vi "Main.vi"() -> ()   [LabVIEW 2019]
doc: "The myRIO Project template acquires acceleration data from the onboard accelerometer and displays the changes of acceleration values in a waveform chart."
uses:
  <vilib>/myRIO/Instrument Drivers/Onboard IO/DIO/typedefs/DIO Reference.ctl
  <vilib>/myRIO/Common/Instrument Driver Framework/Utilities/typedefs/myRIO Generic Hardware Reference.ctl
  <vilib>/myRIO/Common/Instrument Driver Framework/Utilities/typedefs/Hardware Version Enum.ctl
  <vilib>/myRIO/Common/Instrument Driver Framework/Utilities/typedefs/myRIO v1.0 Reference.ctl
  <vilib>/myRIO/Common/Instrument Driver Framework/Utilities/typedefs/Generic FPGA Reference.ctl
  <vilib>/myRIO/Common/Instrument Driver Framework/myRIO v1.0/DIO/typedefs/DIO Channels List.ctl
  <vilib>/myRIO/Common/Instrument Driver Framework/myRIO v1.0/DIO/typedefs/DIO Channels Enum.ctl
  <vilib>/userDefined/High Color/nirio_resource_hc.ctl
  <vilib>/myRIO/Common/Instrument Driver Framework/Utilities/vis/Is FPGA Ref Available.vi
  <vilib>/myRIO/Common/Instrument Driver Framework/myRIO v1.0/DIO/vis/myRIO v1.1 Open DIO.vi
  <vilib>/myRIO/Instrument Drivers/Onboard IO/DIO/vis/Write.vi
  <vilib>/myRIO/Common/Instrument Driver Framework/Utilities/vis/Validate Channels.vi
  <vilib>/myRIO/Common/Instrument Driver Framework/myRIO v1.0/DIO/vis/myRIO v1.0 Reserve DIO.vi
  <vilib>/myRIO/Common/Instrument Driver Framework/myRIO v1.0/UART/vis/myRIO v1.0 Close UART.vi
  <vilib>/myRIO/Common/Instrument Driver Framework/myRIO v1.0/Resource Manager/vis/myRIO v1.0 Reserve Channel List.vi
  <vilib>/myRIO/Common/Instrument Driver Framework/myRIO v1.0/DIO/vis/myRIO v1.0 Build MUX Configuration DIO.vi
  <vilib>/myRIO/Common/Instrument Driver Framework/myRIO v1.0/Resource Manager/vis/myRIO v1.0 Reserve Channel.vi
  <vilib>/myRIO/Common/Instrument Driver Framework/myRIO v1.0/Resource Manager/vis/myRIO v1.0 Unreserve Channel.vi
  <vilib>/myRIO/Common/Instrument Driver Framework/myRIO v1.0/Resource Manager/vis/myRIO v1.0 Create Configuration List.vi
  <vilib>/myRIO/Common/Instrument Driver Framework/myRIO v1.0/Resource Manager/vis/myRIO v1.0 Build Mutex Name.vi
  <vilib>/Utility/VariantDataType/GetNumericInfo.vi
  <vilib>/Utility/error.llb/Error Cluster From Error Code.vi
  <vilib>/myRIO/Common/Instrument Driver Framework/myRIO v1.0/myRIO v1.1 Open.vi
  <vilib>/myRIO/Common/Instrument Driver Framework/Utilities/vis/IO Manager.vi
  <vilib>/myRIO/Common/Instrument Driver Framework/Utilities/vis/Configuration Manager.vi
  <vilib>/myRIO/Common/Instrument Driver Framework/myRIO v1.0/Resource Manager/vis/myRIO v1.0 Configure IO.vi
  <vilib>/myRIO/Common/Instrument Driver Framework/myRIO v1.0/myRIO v1.0 Close.vi
  <vilib>/myRIO/Common/Instrument Driver Framework/myRIO v1.0/DIO/vis/myRIO v1.0 Write DIO.vi
  <vilib>/myRIO/Common/Instrument Driver Framework/Utilities/vis/FPGA Ref Manager.vi
  <vilib>/myRIO/Common/Instrument Driver Framework/myRIO v1.0/myRIO v1.0 Reset FPGA.vi
  <vilib>/myRIO/Common/Instrument Driver Framework/myRIO v1.0/IRQ/vis/myRIO v1.0 IRQ Info FGV.vi
  <vilib>/myRIO/Common/Instrument Driver Framework/myRIO v1.0/IRQ/vis/myRIO v1.0 Timer IRQ Info FGV.vi
  <vilib>/myRIO/Common/Instrument Driver Framework/myRIO v1.0/IRQ/vis/myRIO v1.0 ISR Agent.vi
  <vilib>/myRIO/Instrument Drivers/Utilities/vis/Reset Index.vi
  <vilib>/myRIO/Common/Instrument Driver Framework/myRIO v1.0/Resource Manager/vis/myRIO v1.0 Block Write Resource Manager.vi
  <vilib>/myRIO/Express VI/Onboard IO/DO/DO Express VI.xnode
  <vilib>/myRIO/Instrument Drivers/Onboard IO/DIO/vis/myRIO DIO Open.xnode
  <vilib>/myRIO/Instrument Drivers/Utilities/Utilities.lvlib
  <vilib>/myRIO/Instrument Drivers/Onboard IO/DIO/DIO.lvlib
panel:
  out "Polar Plot":picture
  in  "stop":bool
  in  "seperation factor":i32(slide) scale=1.0..12.0
  in  "Phase Const":i64(slide) scale=0.0..360.0
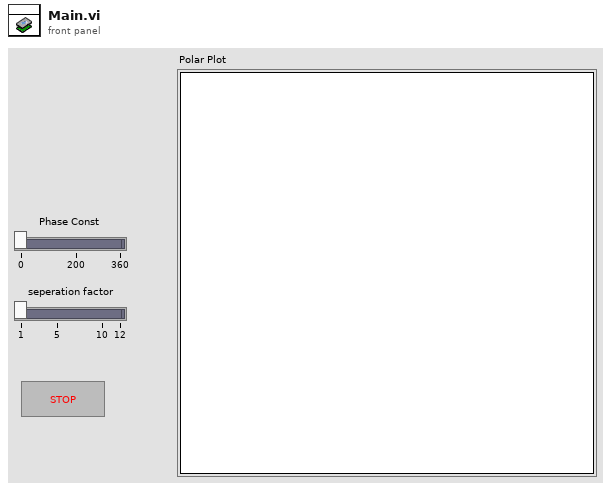
[diagram p1: front panel]
types:
  T1 = typedef "DIO.lvlib/DIO Reference.ctl" = cluster{"myRIO Reference":T2, "DIO Channels List":T6}
  T2 = typedef "myRIO Generic Hardware Reference.ctl" = cluster{"myRIO Model":T3, "myRIO Hardware Reference":T4}
  T3 = typedef "Hardware Version Enum.ctl" = enum16{"Unknown", "myRIO-1900", "myRIO-1950", "roboRIO", "NI ELVIS RIO CM", "ELVIS III"}
  T4 = typedef "myRIO v1.0 Reference.ctl" = cluster{"Generic FPGA Reference":T5, "Allow multiple opens":bool}
  T5 = typedef "Generic FPGA Reference.ctl" = refnum<k20>
  T6 = typedef "DIO Channels List.ctl" = T7[]
  T7 = typedef "DIO Channels Enum.ctl" = enum16{"Not Connected", "C/DIO0", "C/DIO1", "C/DIO2", "C/DIO3", "C/DIO4", "C/DIO5", "C/DIO6", "C/DIO7", "A/DIO0", "A/DIO1", "A/DIO2", "A/DIO3", "A/DIO4", "A/DIO5", "A/DIO6", "A/DIO7", "A/DIO8", "A/DIO9", "A/DIO10", "A/DIO11", "A/DIO12", "A/DIO13", "A/DIO14", "A/DIO15", "A/DIO16", "A/DIO17", "A/DIO18", "A/DIO19", "B/DIO0", "B/DIO1", "B/DIO2", "B/DIO3", "B/DIO4", "B/DIO5", "B/DIO6", "B/DIO7", "B/DIO8", "B/DIO9", "B/DIO10", "B/DIO11", "B/DIO12", "B/DIO13", "B/DIO14", "B/DIO15", "B/DIO16", "B/DIO17", "B/DIO18", "B/DIO19", "LED0", "LED1", "LED2", "LED3", "Button0", "DIO/DIO0", "DIO/DIO1", "DIO/DIO2", "DIO/DIO3", "DIO/DIO4", "DIO/DIO5", "DIO/DIO6", "DIO/DIO7", "DIO/DIO8", "DIO/DIO9", "SPI/CS0", "SPI/CS1", "SPI/CS2", "SPI/CS3", "LED RADIO (Green)", "LED RADIO (Red)", "LED COMM (Green)", "LED COMM (Red)", "LED MODE (Green)", "LED MODE (Red)"}
  T8 = typedef "nirio_resource_hc.ctl" = tag
  T9 = typedef "LVBoundsTypeDef.ctl" = cluster{"Width":u32, "Height":u32}
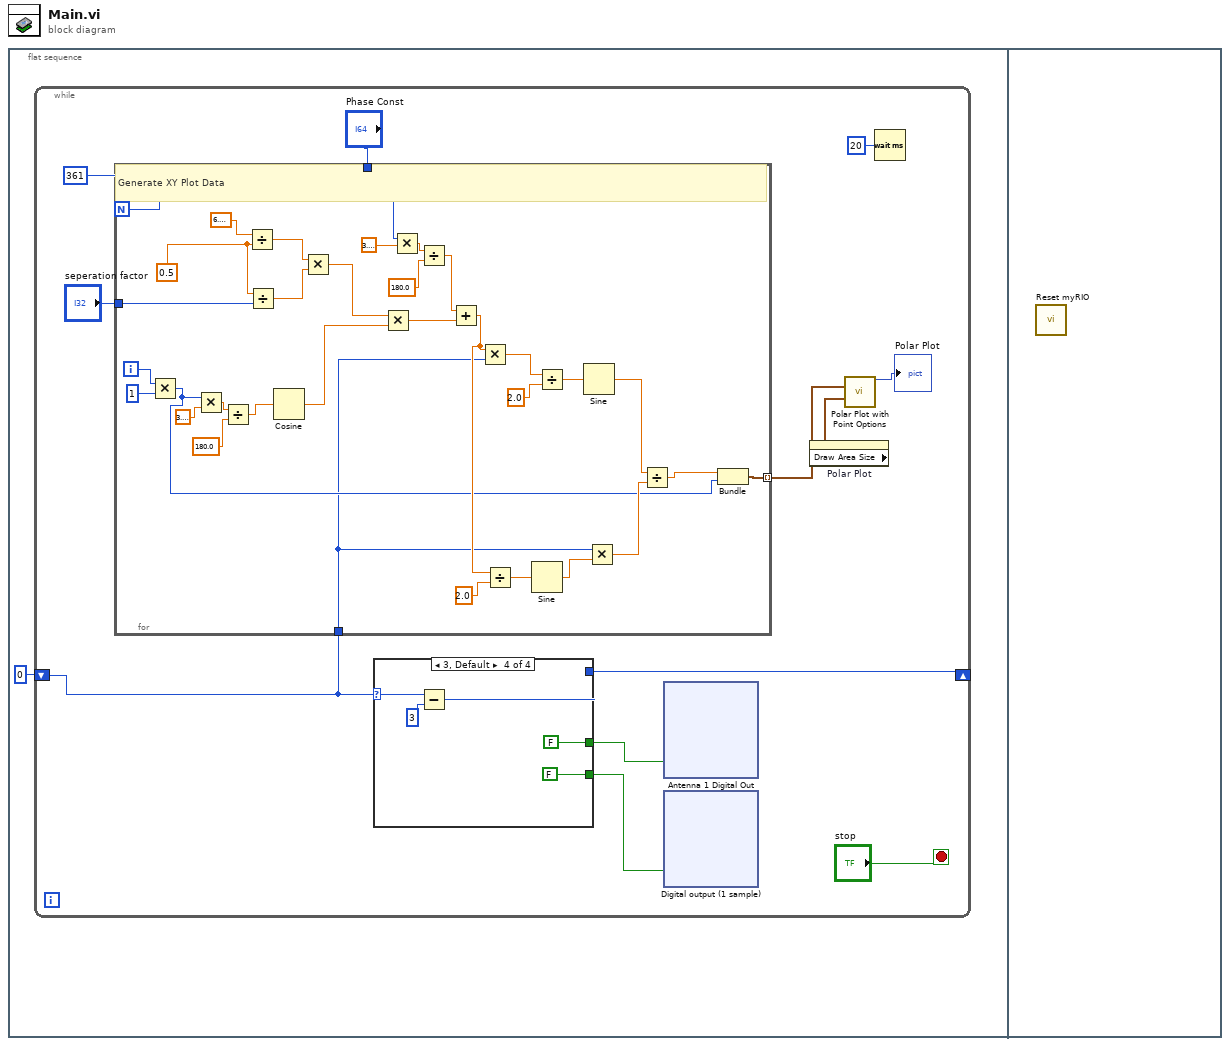
[diagram p0: block diagram]
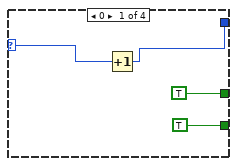
[diagram p2: hidden frame]
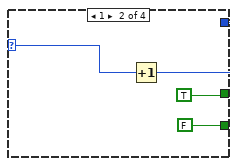
[diagram p3: hidden frame]
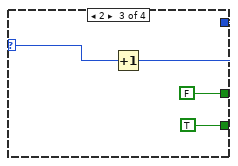
[diagram p4: hidden frame]
diagram:
  n1 = flat-sequence {
    frame #0 {
      n2 = while {
        shift-right: [w7] -> _
        shift-left: 0 -> [w4]
        stop <- "stop" stop-if-true
        n3 = for {
          N: 361 -> [_]
          tunnel: [w113] -> w10 mode=indexing
          tunnel: "seperation factor" -> [w103]
          tunnel: "Phase Const" -> [w102]
          tunnel: w4 -> [w101]
          i -> [w114]
          w122 = 0.5 ("Labda")
          # "Generate XY Plot Data"
          n4 = Multiply(x=w114, y=1) -> (x*y=w104:i32)
          n5 = Multiply(x=w104, y=3.141592653589793) -> (x*y=w126:dbl)
          n6 = Divide(x=w126, y=180.0) -> (x/y=w127:dbl)
          n7 = Divide(x=6.283185307179586, y=w122) -> (x/y=w123:dbl)
          n8 = Divide(x=w122, y=w103) -> (x/y=w124:dbl)
          n9 = Cosine(x=w127) -> (cos(x)=w125:dbl)
          n10 = Multiply(x=w123, y=w124) -> (x*y=w128:dbl)
          n11 = Multiply(x=w128, y=w125) -> (x*y=w131:dbl)
          n12 = Multiply(x=w102, y=3.141592653589793) -> (x*y=w129:dbl)
          n13 = Divide(x=w129, y=180.0) -> (x/y=w130:dbl)
          n14 = Add(x=w130, y=w131) -> (x+y=w105:dbl)
          n15 = Multiply(x=w105, y=w101) -> (x*y=w112:dbl)
          n16 = Divide(x=w105, y=2.0) -> (x/y=w111:dbl)
          n17 = Sine(x=w111) -> (sin(x)=w109:dbl)
          n18 = Divide(x=w112, y=2.0) -> (x/y=w132:dbl)
          n19 = Sine(x=w132) -> (sin(x)=w108:dbl)
          n20 = Multiply(x=w101, y=w109) -> (x*y=w107:dbl)
          n21 = Divide(x=w108, y=w107) -> (x/y=w106:dbl)
          n22 = Bundle(w106, w104) -> (w113:cluster{dbl, i32})  [unwired: 1 in]
        }
        n23 = case shown="3, Default" w4 {
          selector: w4 -> [w87 w91 w95 w100]
          tunnel: [w86 w90 w94 w98] -> w7
          tunnel: [TRUE TRUE FALSE FALSE] -> w3
          tunnel: [TRUE FALSE TRUE FALSE] -> w2
          frame 0 {
            n24 = Increment(x=w87) -> (x+1=w86:i32)
          }
          frame 1 {
            n25 = Increment(x=w91) -> (x+1=w90:i32)
          }
          frame 2 {
            n26 = Increment(x=w95) -> (x+1=w94:i32)
          }
          frame 3, Default {
            n27 = Subtract(x=w100, y=3) -> (x-y=w98:i32)
          }
        }
        n28 = xnode "Antenna 1 Digital Out"("A/DIO0 (Pin 11)"=w3) -> ()  [unwired: 1 in, 1 out]
        n29 = xnode "Digital output (1 sample)"("A/DIO1 (Pin 13)"=w2) -> ()  [unwired: 1 in, 1 out]
        n30 = property on="Polar Plot" class="Pict"() -> ("Draw Area Size"=w11:T9)  [unwired: 2 in, 2 out]
        n31 = call <vilib>:"Polar Plot with Point Options.vi"("data array [mag, phase (deg)]"=w10, "dimensions (w,h)"=w11) -> ("new picture"=→"Polar Plot":picture)  [unwired: 13 in]
        n32 = Wait (ms)(milliseconds to wait=u32 20) -> ()  [unwired: 1 out]
      }
    }
    frame #1 {
      n33 = call <vilib>:"Reset myRIO.vi"() -> ()  [unwired: 11 in, 1 out]
    }
  }
